vi "Graphical Test Runner - Get Version.vi"() -> (1 "Version Info":T1 {"Build Date/Time" format="%<%H:%M:%S\n%d/%m/%Y>T"}, 2 "Dev. Environment?":bool)   [LabVIEW 2011, in "GraphicalTestRunner.lvlib"]
uses:
  GraphicalTestRunner.lvlib
panel:
  # "Copyright © 2007 James Kring, Inc. All rights reserved.\n\nAuthor: Omar Mussa [omar.mussa@jameskring.com]\n\nThis library is provided \"AS IS\" ,WITHOUT WARRANTIES OR \nCONDITIONS OF ANY KIND, either express or implied.\n\nJames Kring, Inc. -- http://www.jameskring.com"
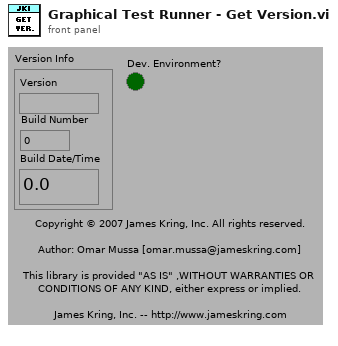
[diagram p1: front panel]
types:
  T1 = cluster{"Version":string, "Build Number":u32, "Build Date/Time":dbl}
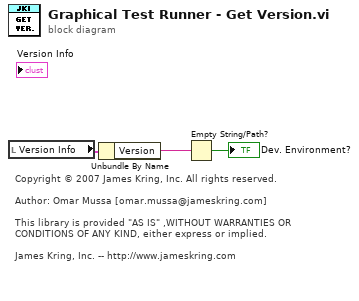
[diagram p0: block diagram]
diagram:
  # "Copyright © 2007 James Kring, Inc. All rights reserved.\n\nAuthor: Omar Mussa [omar.mussa@jameskring.com]\n\nThis library is provided \"AS IS\" ,WITHOUT WARRANTIES OR \nCONDITIONS OF ANY KIND, either express or implied.\n\nJames Kring, Inc. -- http://www.jameskring.com"
  n1 = local read "Version Info"() -> (w2:T1)
  n2 = Unbundle By Name(w2) -> ("Version"=w3:string)
  n3 = Empty String/Path?(string/path=w3) -> (empty?=→"Dev. Environment?":bool)
